vi "CreatePointsOnLine (SubVI).vi"(2 "x values for fit line on plot":dbl[](array[numeric])=[-700.0, -300.0, 100.0, 500.0, 700.0], 10 "intercept":dbl, 11 "slope":dbl) -> (3 "Array":dbl[](array[numeric]))   [LabVIEW 2016]
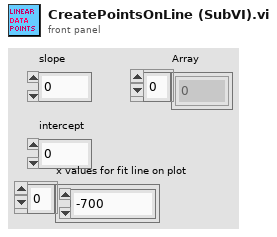
[diagram p1: front panel]
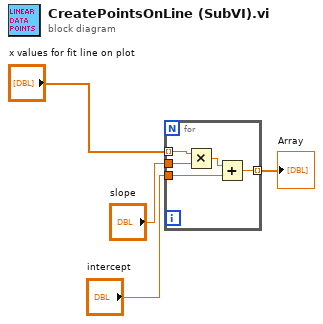
[diagram p0: block diagram]
diagram:
  n1 = for {
    tunnel: "slope" -> [w8]
    tunnel: "intercept" -> [w9]
    tunnel: [w6] -> w3 mode=indexing
    tunnel: "x values for fit line on plot" -> [w5] mode=indexing
    n2 = Multiply(x=w5, y=w8) -> (x*y=w7:dbl)
    n3 = Add(x=w7, y=w9) -> (x+y=w6:dbl)
  }
  "Array" <- w3
